vi "Decode Error.vi"(8 "error in (no error)":errorcluster, 10 "MSS Bit Set (F: No)":bool, 11 "VISA resource name":refnum<visa-resource-name>) -> (0 "error out":errorcluster, 2 "Error Message":string, 3 "VISA resource name out":refnum<visa-resource-name>)   [LabVIEW 2020, in "Lake Shore 336.lvlib"]
doc: "This VI is designed to be called by the 336 Error Query VI. It's function is to query the 336 Status Byte and decode errors if the Status Byte reports errors are present. \n\nNote that the calling VI checks the Status Byte in the case of a timeout error. If the calling VI indicates the Status Byte is already reporting errors, this VI will not query the Status Byte again, it will go straight to the process of decoding errors.\n\nThe following conditions will be returned as errors in the Error Out cluster:\n<B>Processor Communication Error</B>\n<B>Query Error</B>\n<B>Execution Error</B>\n<B>Command Error</B>\n<B>Calibration Error</B>\n\nThe following conditions will be returned as warnings in the Error Out cluster:\n<B>Sensor Alarming</B>\n<B>Invalid Reading</B>\n<B>Temperature Underrange</B>\n<B>Temperature Overrange</B>\n<B>Sensor Units Zero</B>\n<B>Sensor Units Overrange</B>"
uses:
  Lake Shore 336.lvlib
  Instance           1 20Saved   Decode Error .vi
  Instance           2 20Saved   Decode Error .vi
  Instance           3 20Saved   Decode Error .vi
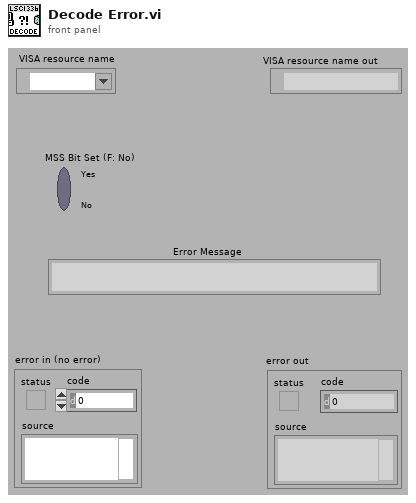
[diagram p1: front panel]
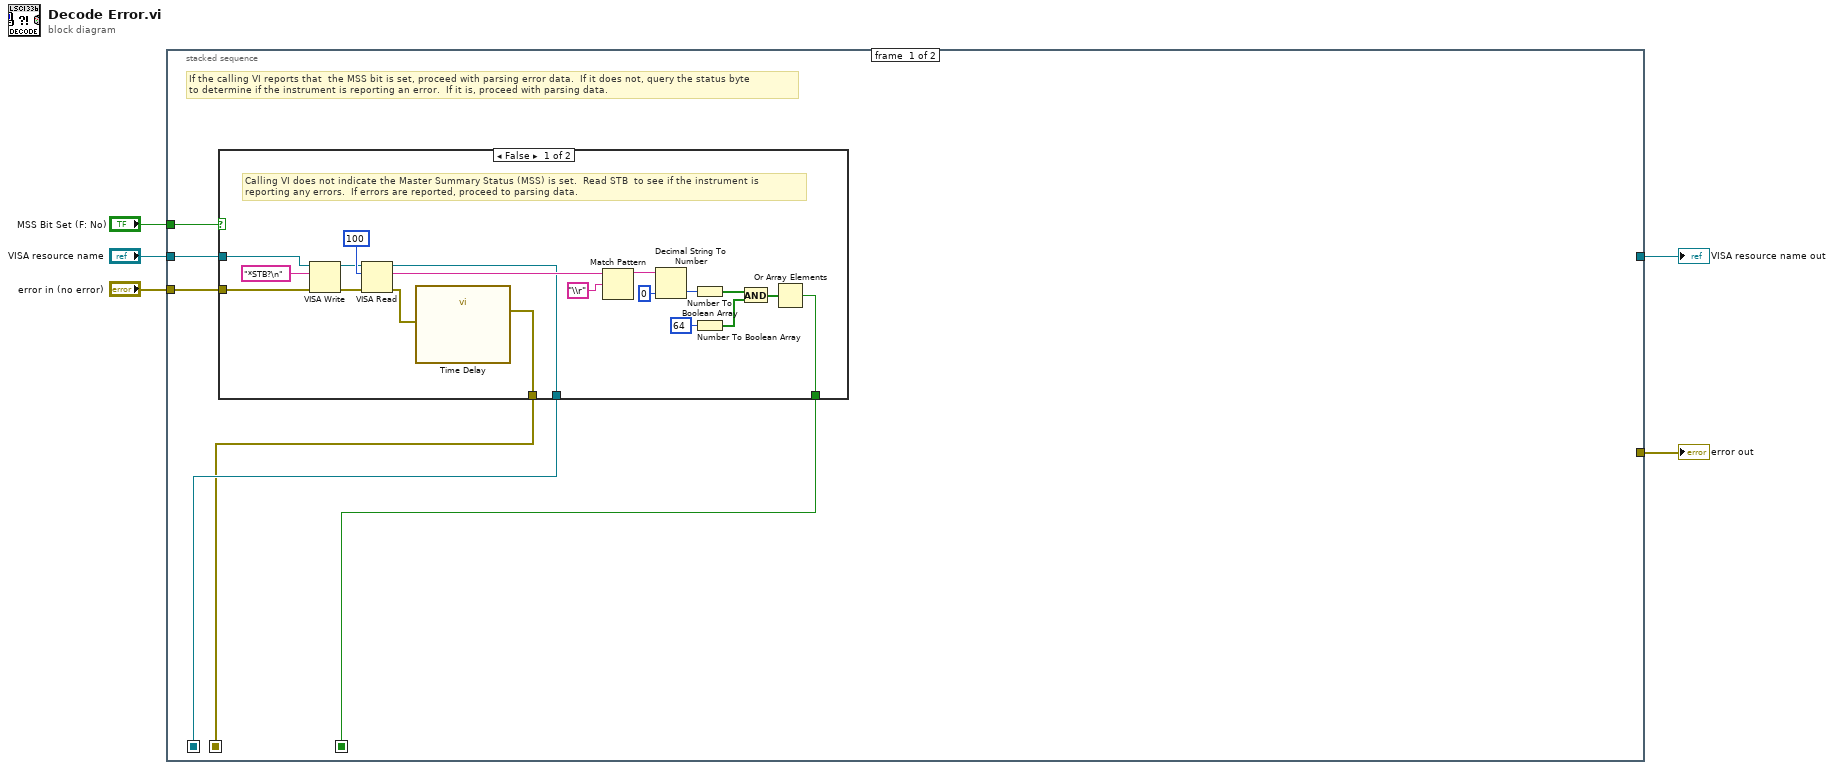
[diagram p0: block diagram]
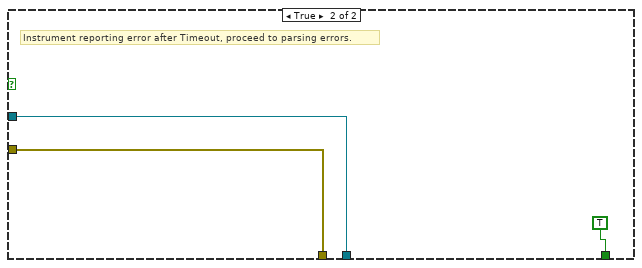
[diagram p2: hidden frame]
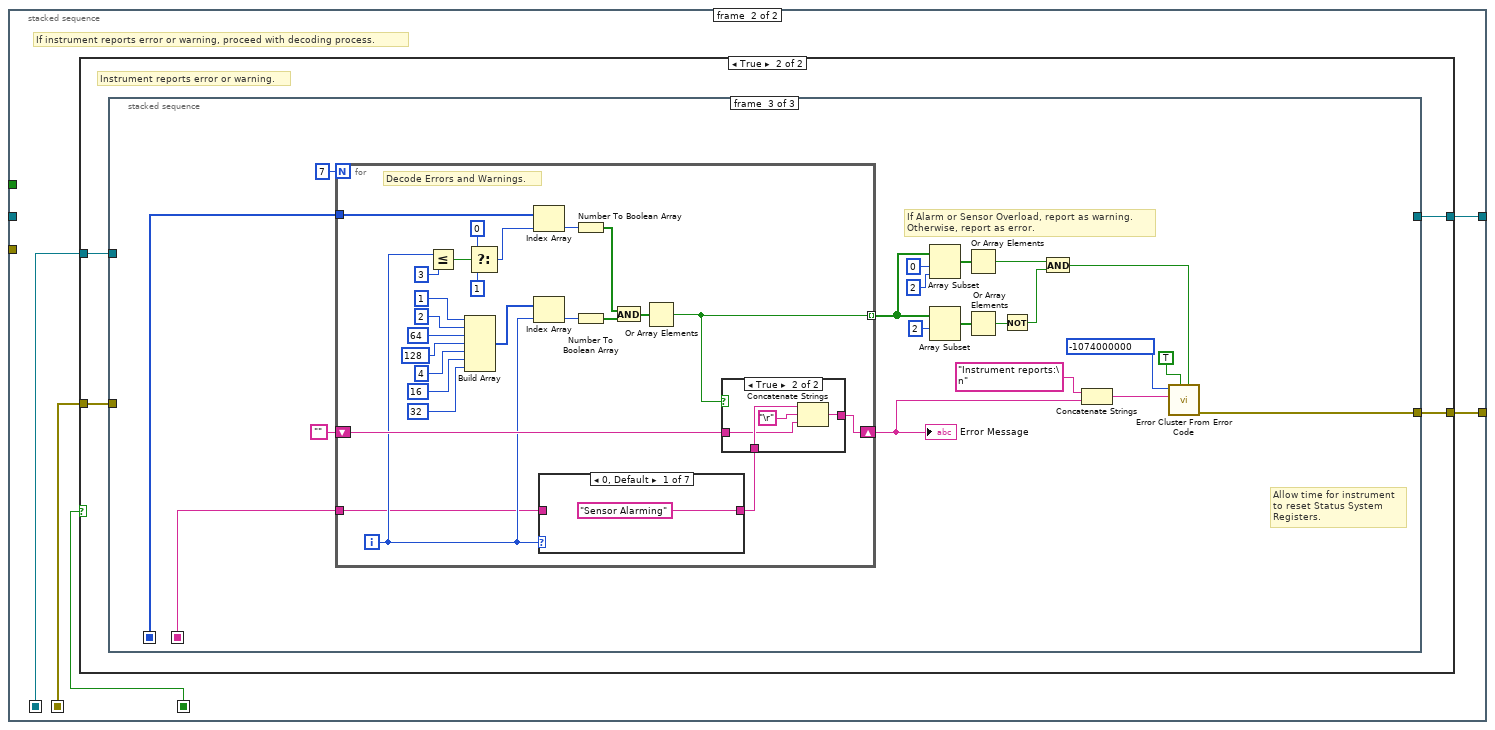
[diagram p3: hidden frame]
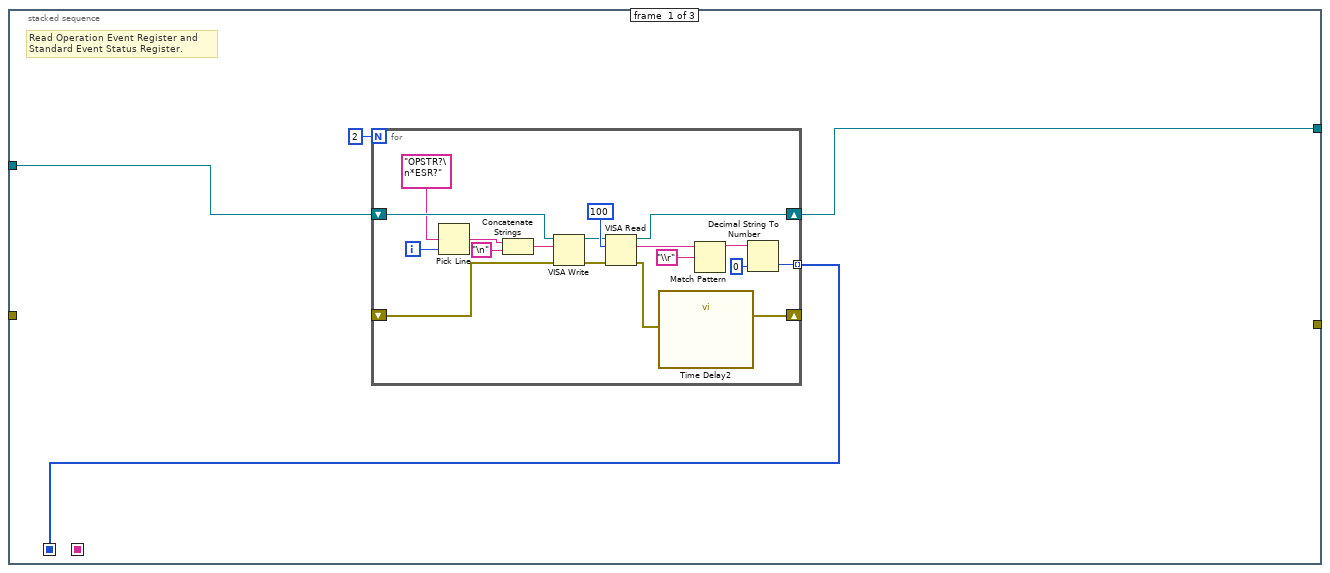
[diagram p5: hidden frame]
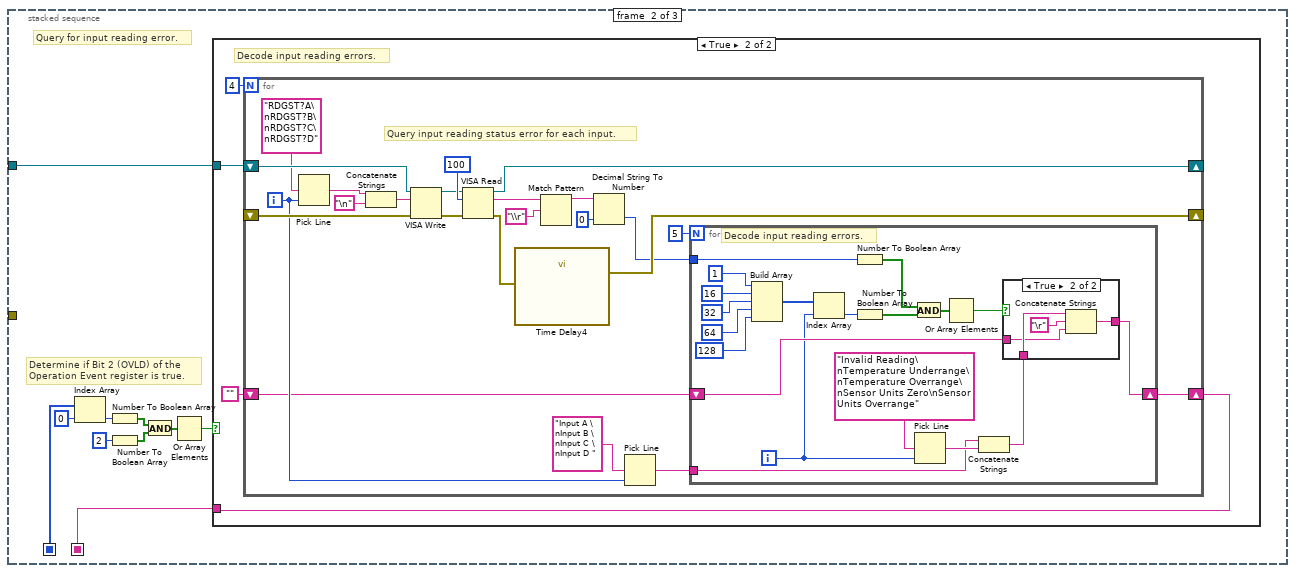
[diagram p6: hidden frame]
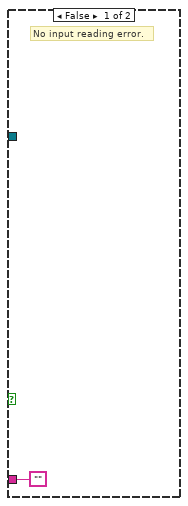
[diagram p7: hidden frame]
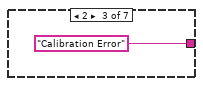
[diagram p10: hidden frame]
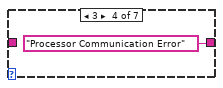
[diagram p11: hidden frame]
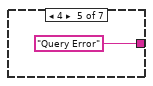
[diagram p12: hidden frame]
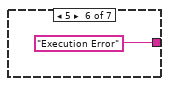
[diagram p13: hidden frame]
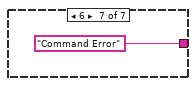
[diagram p14: hidden frame]
diagram:
  n1 = stacked-sequence {
    seq-local: [w8 _] -> [_ w34]
    seq-local: [w7 _] -> [_ w38]
    seq-local: [w6 _] -> [_ w37]
    tunnel: "MSS Bit Set (F: No)" -> [w11 _]
    tunnel: "VISA resource name" -> [w10 _]
    tunnel: "error in (no error)" -> [w9 _]
    tunnel: [_ w36] -> w5
    tunnel: [_ w35] -> w4
    frame #0 {
      # "If the calling VI reports that  the MSS bit is set, proceed with parsing error data.  If it does not, query the status byte\nto determine if the instrument is reporting an error.  If it is, proceed with parsing data."
      n2 = case shown="False" w11 {
        tunnel: w10 -> [w13 w32]
        tunnel: w9 -> [w12 w33]
        tunnel: [w18 TRUE] -> w8
        tunnel: [w14 w33] -> w6
        tunnel: [w17 w32] -> w7
        frame False {
          # "Calling VI does not indicate the Master Summary Status (MSS) is set.  Read STB  to see if the instrument is\nreporting any errors.  If errors are reported, proceed to parsing data."
          n3 = VISA Write(VISA resource name=w13, write buffer="*STB?\n", error in (no error)=w12) -> (VISA resource name out=w28:refnum<visa-resource-name>, error out=w27:errorcluster)  [unwired: 1 out]
          n4 = VISA Read(VISA resource name=w28, byte count=100, error in (no error)=w27) -> (VISA resource name out=w17:refnum<visa-resource-name>, read buffer=w30:string, error out=w15:errorcluster)  [unwired: 1 out]
          n5 = call "Time Delay"("error in (no error)"=w15) -> ("error out"=w14:errorcluster)  [unwired: 10 in]
          n6 = Match Pattern(string=w30, regular expression="\\r") -> (before substring=w23:string)  [unwired: 1 in, 3 out]
          n7 = Decimal String To Number(string=w23, default (0L)=u16 0) -> (number=w16:u16)  [unwired: 1 in, 1 out]
          n8 = Number To Boolean Array(number=w16) -> (Boolean array=w19:bool[])
          n9 = Number To Boolean Array(number=64) -> (Boolean array=w21:bool[])
          n10 = And(x=w19, y=w21) -> (x .and. y?=w20:bool[])
          n11 = Or Array Elements(Boolean array=w20) -> (logical OR=w18:bool)
        }
        frame True {
          # "Instrument reporting error after Timeout, proceed to parsing errors."
        }
      }
    }
    frame #1 {
      # "If instrument reports error or warning, proceed with decoding process."
      n12 = case shown="True" w34 {
        tunnel: w38 -> [w40 w44]
        tunnel: w37 -> [w39 w43]
        tunnel: [w40 w42] -> w36
        tunnel: [w39 w41] -> w35
        frame False {
          # "No instrument error or warning reported."
        }
        frame True {
          # "Instrument reports error or warning."
          n13 = stacked-sequence {
            seq-local: [w45 _ _] -> [_ w75 w132]
            seq-local: [_ w68 _] -> [_ _ w130]
            tunnel: w44 -> [w47 w69 _]
            tunnel: w43 -> [_ _ _]
            tunnel: [w46 _ _] -> w42
            tunnel: [_ _ w129] -> w41
            frame #0 {
              # "Read Operation Event Register and \nStandard Event Status Register."
              n14 = for {
                N: 2 -> [_]
                shift-right: [w64] -> w46
                shift-left: w47 -> [w65]
                shift-right: [w52] -> _
                shift-left: _ -> [w54]
                tunnel: [w55] -> w45 mode=indexing
                i -> [w66]
                n15 = Pick Line(multi-line string="OPSTR?\n*ESR?", line index=w66) -> (output string=w50:string)  [unwired: 1 in]
                n16 = Concatenate Strings(w50, "\n") -> (w49:string)
                n17 = VISA Write(VISA resource name=w65, write buffer=w49, error in (no error)=w54) -> (VISA resource name out=w61:refnum<visa-resource-name>, error out=w60:errorcluster)  [unwired: 1 out]
                n18 = VISA Read(VISA resource name=w61, byte count=100, error in (no error)=w60) -> (VISA resource name out=w64:refnum<visa-resource-name>, read buffer=w63:string, error out=w53:errorcluster)  [unwired: 1 out]
                n19 = call "Time Delay2"("error in (no error)"=w53) -> ("error out"=w52:errorcluster)  [unwired: 10 in]
                n20 = Match Pattern(string=w63, regular expression="\\r") -> (before substring=w57:string)  [unwired: 1 in, 3 out]
                n21 = Decimal String To Number(string=w57, default (0L)=u16 0) -> (number=w55:u16)  [unwired: 1 in, 1 out]
              }
            }
            frame #1 {
              # "Query for input reading error."
              # "Determine if Bit 2 (OVLD) of the \nOperation Event register is true."
              n22 = Index Array(array=w75, index=0) -> (element=w76:u16)
              n23 = Number To Boolean Array(number=w76) -> (Boolean array=w71:bool[])
              n24 = Number To Boolean Array(number=2) -> (Boolean array=w70:bool[])
              n25 = And(x=w71, y=w70) -> (x .and. y?=w72:bool[])
              n26 = Or Array Elements(Boolean array=w72) -> (logical OR=w67:bool)
              n27 = case shown="True" w67 {
                tunnel: w69 -> [_ w80]
                tunnel: ["" w78] -> w68
                frame False {
                  # "No input reading error."
                }
                frame True {
                  # "Decode input reading errors."
                  n28 = for {
                    N: 4 -> [_]
                    shift-right: [w103] -> _
                    shift-left: w80 -> [w104]
                    shift-right: [w93] -> _
                    shift-left: _ -> [w95]
                    shift-right: [w82] -> w78
                    shift-left: "" -> [w83]
                    i -> [w87]
                    # "Query input reading status error for each input."
                    n29 = Pick Line(multi-line string="RDGST?A\nRDGST?B\nRDGST?C\nRDGST?D", line index=w87) -> (output string=w91:string)  [unwired: 1 in]
                    n30 = Concatenate Strings(w91, "\n") -> (w90:string)
                    n31 = VISA Write(VISA resource name=w104, write buffer=w90, error in (no error)=w95) -> (VISA resource name out=w100:refnum<visa-resource-name>, error out=w99:errorcluster)  [unwired: 1 out]
                    n32 = VISA Read(VISA resource name=w100, byte count=100, error in (no error)=w99) -> (VISA resource name out=w103:refnum<visa-resource-name>, read buffer=w102:string, error out=w94:errorcluster)  [unwired: 1 out]
                    n33 = call "Time Delay4"("error in (no error)"=w94) -> ("error out"=w93:errorcluster)  [unwired: 10 in]
                    n34 = Match Pattern(string=w102, regular expression="\\r") -> (before substring=w96:string)  [unwired: 1 in, 3 out]
                    n35 = Decimal String To Number(string=w96, default (0L)=u16 0) -> (number=w85:u16)  [unwired: 1 in, 1 out]
                    n36 = Pick Line(multi-line string="Input A \nInput B \nInput C \nInput D ", line index=w87) -> (output string=w84:string)  [unwired: 1 in]
                    n37 = for {
                      N: 5 -> [_]
                      tunnel: w85 -> [w117]
                      tunnel: w84 -> [w115]
                      shift-right: [w113] -> w82
                      shift-left: w83 -> [w108]
                      i -> [w107]
                      # "Decode input reading errors."
                      n38 = Build Array(1, 16, 32, 64, 128) -> (w106:i32[])
                      n39 = Index Array(array=w106, index=w107) -> (element=w120:i32)
                      n40 = Number To Boolean Array(number=w117) -> (Boolean array=w121:bool[])
                      n41 = Number To Boolean Array(number=w120) -> (Boolean array=w123:bool[])
                      n42 = And(x=w121, y=w123) -> (x .and. y?=w122:bool[])
                      n43 = Pick Line(multi-line string="Invalid Reading\nTemperature Underrange\nTemperature Overrange\nSensor Units Zero\nSensor Units Overrange", line index=w107) -> (output string=w116:string)  [unwired: 1 in]
                      n44 = Or Array Elements(Boolean array=w122) -> (logical OR=w118:bool)
                      n45 = Concatenate Strings(w115, w116) -> (w114:string)
                      n46 = case shown="True" w118 {
                        tunnel: w108 -> [w124 w125]
                        tunnel: w114 -> [_ w128]
                        tunnel: [w124 w127] -> w113
                        frame False {
                        }
                        frame True {
                          n47 = Concatenate Strings(w128, "\r", w125) -> (w127:string)
                        }
                      }
                    }
                  }
                }
              }
            }
            frame #2 {
              # "Allow time for instrument\nto reset Status System\nRegisters."
              # "If Alarm or Sensor Overload, report as warning.\nOtherwise, report as error."
              n48 = for {
                N: 7 -> [_]
                shift-right: [w157] -> w146
                shift-left: "" -> [w158]
                tunnel: w132 -> [w167]
                tunnel: [w159] -> w141 mode=indexing
                tunnel: w130 -> [w150]
                i -> [w152]
                # "Decode Errors and Warnings."
                n49 = Less Or Equal?(x=w152, y=3) -> (x <= y?=w166:bool)
                n50 = Build Array(1, 2, 64, 128, 4, 16, 32) -> (w170:i32[])
                n51 = Select(t=0, s=w166, f=1) -> (s? t:f=w163:i32)
                n52 = Index Array(array=w167, index=w163) -> (element=w162:u16)
                n53 = Index Array(array=w170, index=w152) -> (element=w169:i32)
                n54 = case shown="0, Default" w152 {
                  tunnel: ["Sensor Alarming" w175 "Calibration Error" "Processor Communication Error" "Query Error" "Execution Error" "Command Error"] -> w151
                  tunnel: w150 -> [_ w175 _ _ _ _ _]
                  frame 0, Default {
                  }
                  frame 1 {
                  }
                  frame 2 {
                  }
                  frame 3 {
                  }
                  frame 4 {
                  }
                  frame 5 {
                  }
                  frame 6 {
                  }
                }
                n55 = Number To Boolean Array(number=w162) -> (Boolean array=w171:bool[])
                n56 = Number To Boolean Array(number=w169) -> (Boolean array=w173:bool[])
                n57 = And(x=w171, y=w173) -> (x .and. y?=w172:bool[])
                n58 = Or Array Elements(Boolean array=w172) -> (logical OR=w159:bool)
                n59 = case shown="True" w159 {
                  tunnel: w158 -> [w181 w182]
                  tunnel: w151 -> [_ w185]
                  tunnel: [w181 w184] -> w157
                  frame False {
                  }
                  frame True {
                    n60 = Concatenate Strings(w185, "\r", w182) -> (w184:string)
                  }
                }
              }
              "Error Message" <- w146
              n61 = Array Subset(array=w141, index=0, length=2) -> (w139:bool[])
              n62 = Array Subset(array=w141, index=2) -> (w138:bool[])  [unwired: 1 in]
              n63 = Or Array Elements(Boolean array=w139) -> (logical OR=w137:bool)
              n64 = Or Array Elements(Boolean array=w138) -> (logical OR=w136:bool)
              n65 = Not(x=w136) -> (.not. x?=w135:bool)
              n66 = And(x=w137, y=w135) -> (x .and. y?=w133:bool)
              n67 = Concatenate Strings("Instrument reports:\n" ("Source"), w146) -> (w143:string)
              n68 = call <vilib>:"Error Cluster From Error Code.vi"("is warning? (False)"=w133, "show call chain? (False)"=TRUE, "error message (\"\")"=w143, "error code (0)"=-1074000000 ("Code")) -> ("error out"=w129:errorcluster)  [unwired: 5 in]
            }
          }
        }
      }
    }
  }
  "error out" <- w4
  "VISA resource name out" <- w5
